vi "报文解析.vi"(9 "长度":i32, 10 "起始位":i32, 11 "MessageBuffer":T1) -> (3 "数字":u32)   [LabVIEW 2020]
panel:
  out "MessageBuffer 2":T1 {"ID" format="%.0x"}
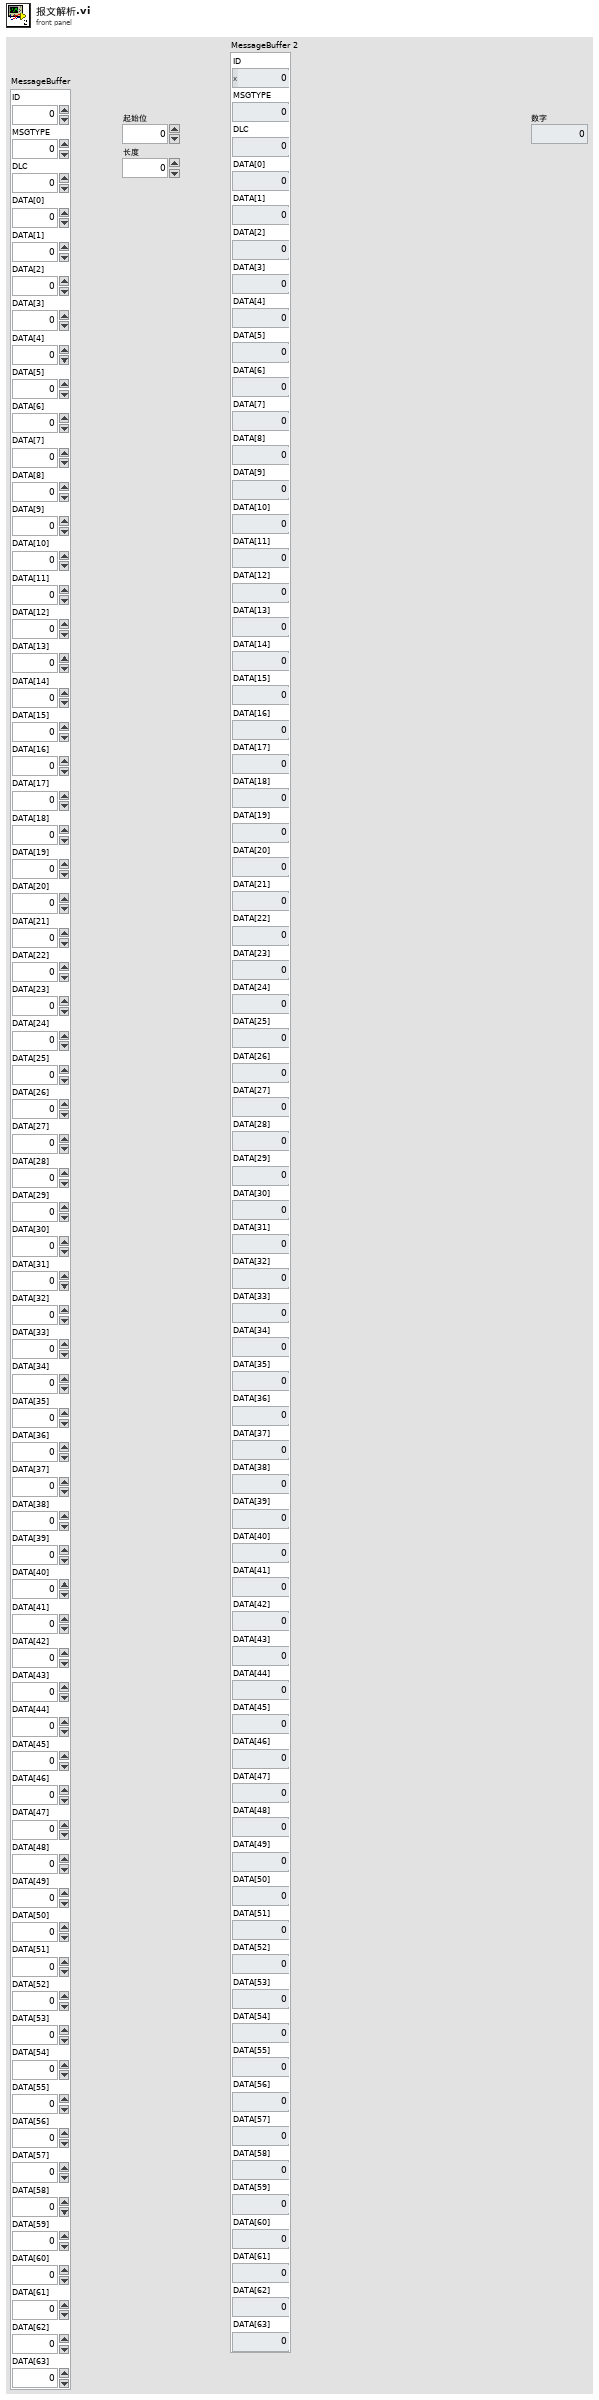
[diagram p1: front panel]
types:
  T1 = cluster{"ID":u32, "MSGTYPE":u8, "DLC":u8, "DATA[0]":u8, "DATA[1]":u8, "DATA[2]":u8, "DATA[3]":u8, "DATA[4]":u8, "DATA[5]":u8, "DATA[6]":u8, "DATA[7]":u8, "DATA[8]":u8, "DATA[9]":u8, "DATA[10]":u8, "DATA[11]":u8, "DATA[12]":u8, "DATA[13]":u8, "DATA[14]":u8, "DATA[15]":u8, "DATA[16]":u8, "DATA[17]":u8, "DATA[18]":u8, "DATA[19]":u8, "DATA[20]":u8, "DATA[21]":u8, "DATA[22]":u8, "DATA[23]":u8, "DATA[24]":u8, "DATA[25]":u8, "DATA[26]":u8, "DATA[27]":u8, "DATA[28]":u8, "DATA[29]":u8, "DATA[30]":u8, "DATA[31]":u8, "DATA[32]":u8, "DATA[33]":u8, "DATA[34]":u8, "DATA[35]":u8, "DATA[36]":u8, "DATA[37]":u8, "DATA[38]":u8, "DATA[39]":u8, "DATA[40]":u8, "DATA[41]":u8, "DATA[42]":u8, "DATA[43]":u8, "DATA[44]":u8, "DATA[45]":u8, "DATA[46]":u8, "DATA[47]":u8, "DATA[48]":u8, "DATA[49]":u8, "DATA[50]":u8, "DATA[51]":u8, "DATA[52]":u8, "DATA[53]":u8, "DATA[54]":u8, "DATA[55]":u8, "DATA[56]":u8, "DATA[57]":u8, "DATA[58]":u8, "DATA[59]":u8, "DATA[60]":u8, "DATA[61]":u8, "DATA[62]":u8, "DATA[63]":u8}
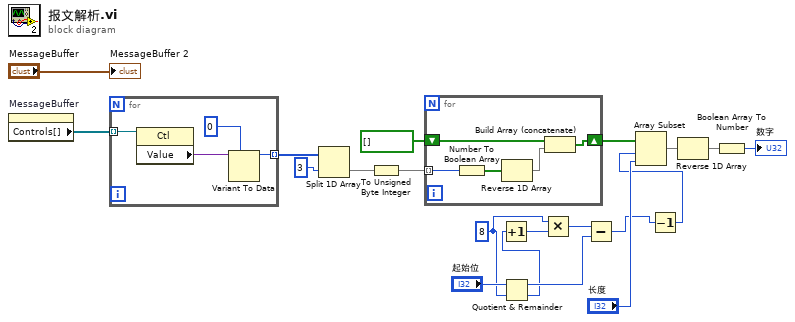
[diagram p0: block diagram]
diagram:
  w3 = 8 ("y")
  n1 = property on="MessageBuffer" class="Clust (严格)"() -> ("Controls[]"=w20:refnum<vi>[])  [unwired: 2 in, 2 out]
  n2 = for {
    tunnel: w20 -> [w24] mode=indexing
    tunnel: [w21] -> w19 mode=indexing
    n3 = property class="Ctl"(reference=w24) -> ("Value"=w23:variant)  [unwired: 1 in, 2 out]
    n4 = Variant To Data(type=u8 0, Variant=w23) -> (data=w21:u8)  [unwired: 1 in, 1 out]
  }
  n5 = Split 1D Array(array=w19, index=3 ("索引")) -> (second subarray=w13:u8[])  [unwired: 1 out]
  n6 = To Unsigned Byte Integer(number=w13) -> (unsigned 8bit integer=w12:u8[])
  n7 = for {
    shift-right: [w29] -> w16
    shift-left: bool[] [] -> [w28]
    tunnel: w12 -> [w27] mode=indexing
    n8 = Number To Boolean Array(number=w27) -> (Boolean array=w26:bool[])
    n9 = Reverse 1D Array(array=w26) -> (reversed array=w25:bool[])
    n10 = Build Array (concatenate)(w28, w25) -> (w29:bool[])
  }
  n11 = Quotient & Remainder(x="起始位", y=w3) -> (x-y*floor(x/y)=w6:i32, floor(x/y)=w4:i32)
  n12 = Increment(x=w4) -> (x+1=w5:i32)
  n13 = Multiply(x=w3, y=w5) -> (x*y=w7:i32)
  n14 = Subtract(x=w7, y=w6) -> (x-y=w2:i32)
  n15 = Decrement(x=w2) -> (x-1=w1:i32)
  n16 = Array Subset(array=w16, index=w1, length="长度") -> (w10:bool[])
  n17 = Reverse 1D Array(array=w10) -> (reversed array=w9:bool[])
  n18 = Boolean Array To Number(Boolean array=w9) -> (number=→"数字":u32)
  "MessageBuffer 2" <- "MessageBuffer"
